vi "test.vi"() -> ()   [LabVIEW 2020]
uses:
  <vilib>/rvi/Emulation/niFpgaGetClockAttributes.vi
  <vilib>/rvi/Emulation/niFpgaSctlEmulationGetInTimedLoop.vi
  <vilib>/rvi/Emulation/niFpgaEmulationReportErrorSimple.vi
  <vilib>/rvi/DataTransferAndStorage/Container/Common/niFpgaContainerExecOnDevCompGetState.vi
  <vilib>/rvi/Emulation/niFpgaEmulationIsFPGAContextNoSignature.vi
  <vilib>/rvi/DataTransferAndStorage/Container/Common/niFpgaContainerGetUniqueNameForEmu.vi
  <vilib>/rvi/Memory/Memory_Emulation/niFpgaMemoryEmulationCacheClearOnFirstRun.vi
  <vilib>/rvi/Memory/Memory_Emulation/nirvimemoryEmulationManagerCache_MakeExclusive.vi
  <vilib>/rvi/Memory/Memory_Emulation/niFpgaMemoryEmulationValidateCache.vi
  <vilib>/rvi/Memory/Memory_Emulation/nirvimemoryEmulationManagerCache_InsertValue.vi
  <vilib>/Utility/error.llb/Clear Errors.vi
  <vilib>/rvi/Memory/Memory_Emulation/nirvimemoryEmulationManagerCache_ReleaseExclusive.vi
  <vilib>/rvi/Memory/Memory_Emulation/nirvimemoryEmulationManagerCache_GetValue.vi
  <vilib>/rvi/Memory/Memory_Emulation/nirvimemoryEmulationManagerCache_SetValue.vi
  <vilib>/rvi/Emulation/niFpgaProcessEmulError.vi
  <vilib>/rvi/DataTransferAndStorage/Container/Common/niFpgaContainerSetEmuInfo.vi
  <vilib>/rvi/eio/common/nirviEmuReportErrorAndStop.vi
  <vilib>/rvi/interface/RandomDataEmulation/niFpgaRandomDataHandleErrors.vi
  <vilib>/rvi/errors/niFpgaSetErrorForExecOnDevCompSimple.vi
  <vilib>/rvi/FIFO/Fifo_Resource/nirvififoEmulationSetSize.vi
  <vilib>/rvi/FIFO/Fifo_Resource/nirviFifoEmulationQueueMgr.vi
  <instcachedir>/0/nirviFifoEmulationQueueMgr_E5CAEC123FF24DC58D834DCA3CDAA9B5.lvgen/nirviFifoEmulationQueueMgr_E5CAEC123FF24DC58D834DCA3CDAA9B5_004.vi
  <vilib>/rvi/FIFO/Fifo_Resource/nirvififoEmulationDetermineInputValidOut.vi
  <vilib>/rvi/FIFO/Fifo_Resource/nirvififoEmulationCreateLock.vi
  <vilib>/rvi/FIFO/Fifo_Resource/nirvififoEmulationObtainLock.vi
  <vilib>/rvi/FIFO/Fifo_Resource/nirvififoEmulationReleaseLock.vi
  <vilib>/rvi/occurrence/nirviWaitOnOccurrenceBase.vi
  <vilib>/rvi/errors/nirviReportUnexpectedCaseInternalError.vi
  <vilib>/rvi/errors/nirviReportUnexpectedCaseInternalError (U32).vi
  <vilib>/rvi/Emulation/niFpgaSctlEmulationResourceMgr.vi
  <vilib>/rvi/Emulation/niFpgaCriticalErrorInLSC.vi
  <vilib>/rvi/DataTransferAndStorage/Container/XNode/niFpgaContainer.xnode
  <vilib>/rvi/DataTransferAndStorage/Register/Emulation/niFpgaRegisterEmulationRefIn.vi
  <vilib>/rvi/LocalResourceManager/LocalResourceManager.xnode
  <vilib>/rvi/interface/RandomDataEmulation/nirviRandomDataFpgaReadWriteTemplate.vi
  <vilib>/rvi/FIFO/Fifo_Resource/niFpgaFifoEmulationRefIn.vi
  <vilib>/rvi/Memory/Memory_Emulation/niFpgaMemoryEmulationRefIn.vi
  <vilib>/eio/EIONode/EIONode.xnode
  <vilib>/rvi/eio/common/nirviEmuTemplateMethod_errors.vi
panel:
  out "Actual loop rate (ticks) 3":u32
  out "Timed Out? 4":bool
  out "Mod1/AI0 4":fxp<+/-,32,16>
  out "data read iteration":i32
  out "Actual loop rate (ticks) 2":u32
  out "Timed Out? 3":bool
  out "Mod1/AI0 3":fxp<+/-,32,16>
  out "array w/ subset deleted 2":fxp<+/-,32,16>[](array[numeric])
  out "fixed-point":fxp<+/-,32,16>
  out "fixed-point 2":fxp<+/-,32,16>
  out "loop number":i32
  out "x > y?":bool
  in  "stop target":bool
  out "array w/ subset deleted":fxp<+/-,32,16>[](array[numeric])
  out "y(MLP1)":fxp<+/-,32,16>
  out "y(MLP2)":fxp<+/-,32,16>
  out "Timed Out? 2":bool
  out "Mod1/AI0 2":fxp<+/-,32,16>
  out "Actual loop rate (ticks)":u32
  out "Timed Out?":bool
  out "Mod1/AI0":fxp<+/-,32,16>
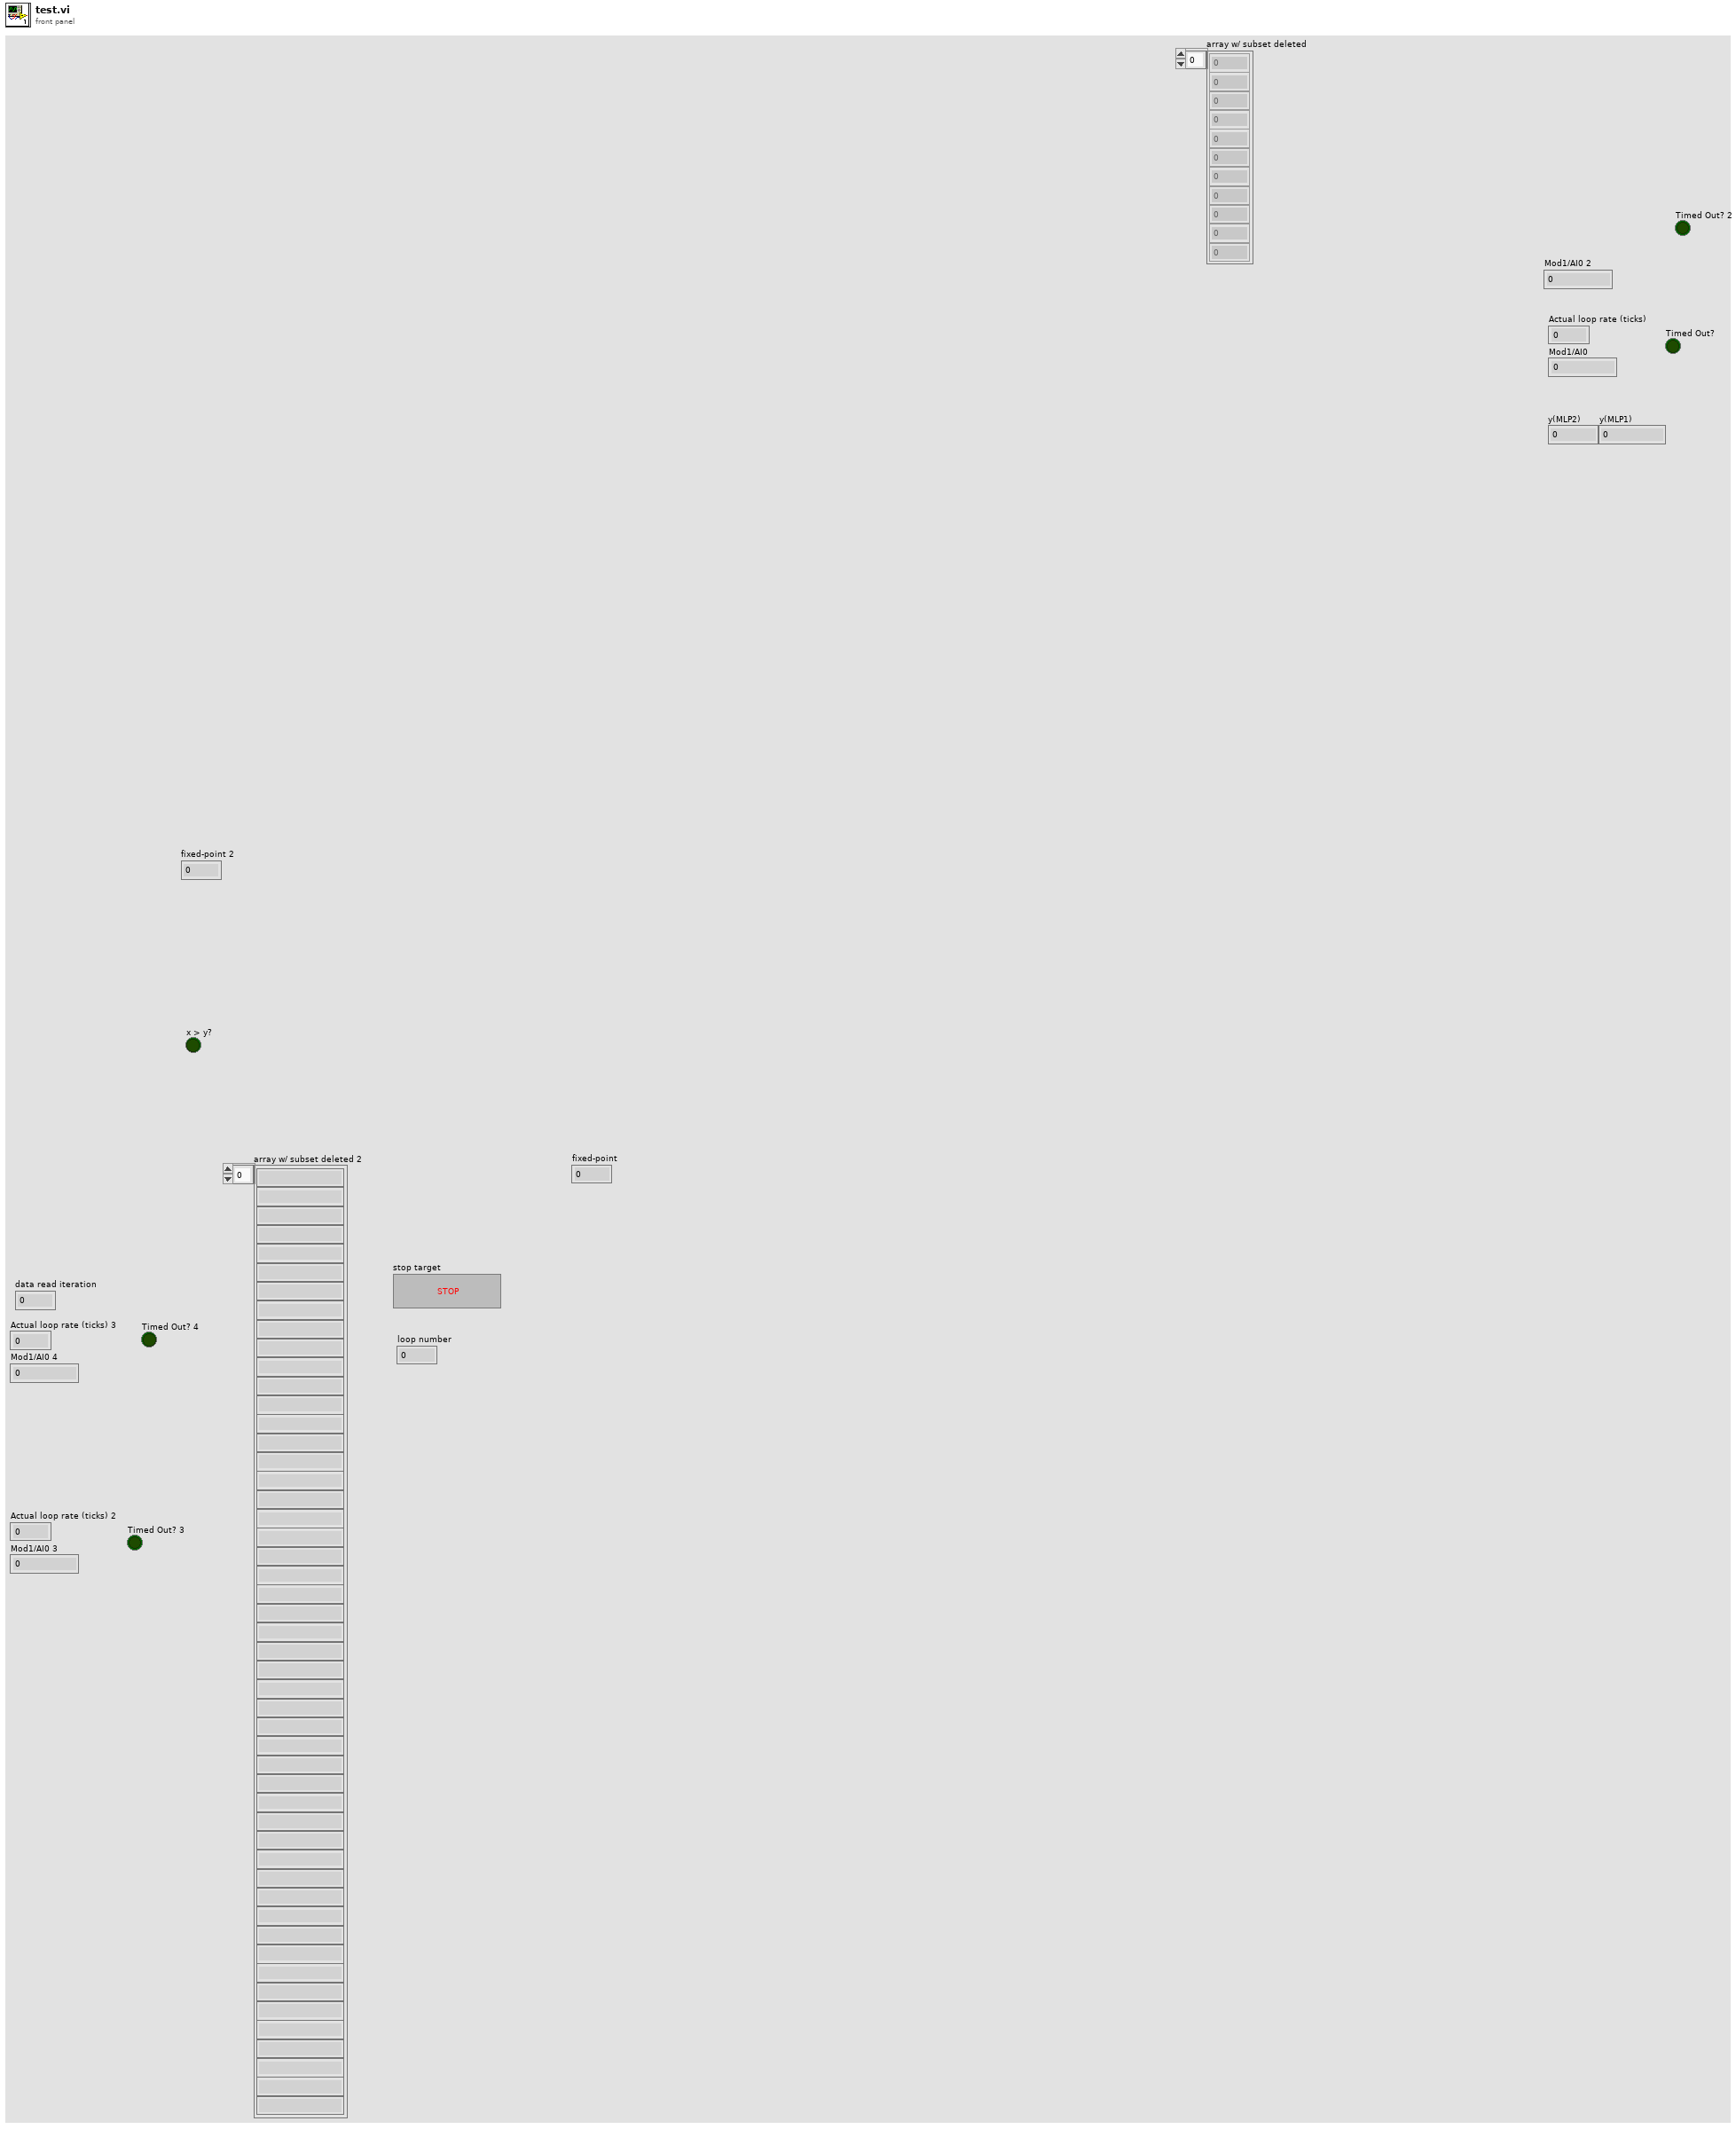
[diagram p1: front panel]
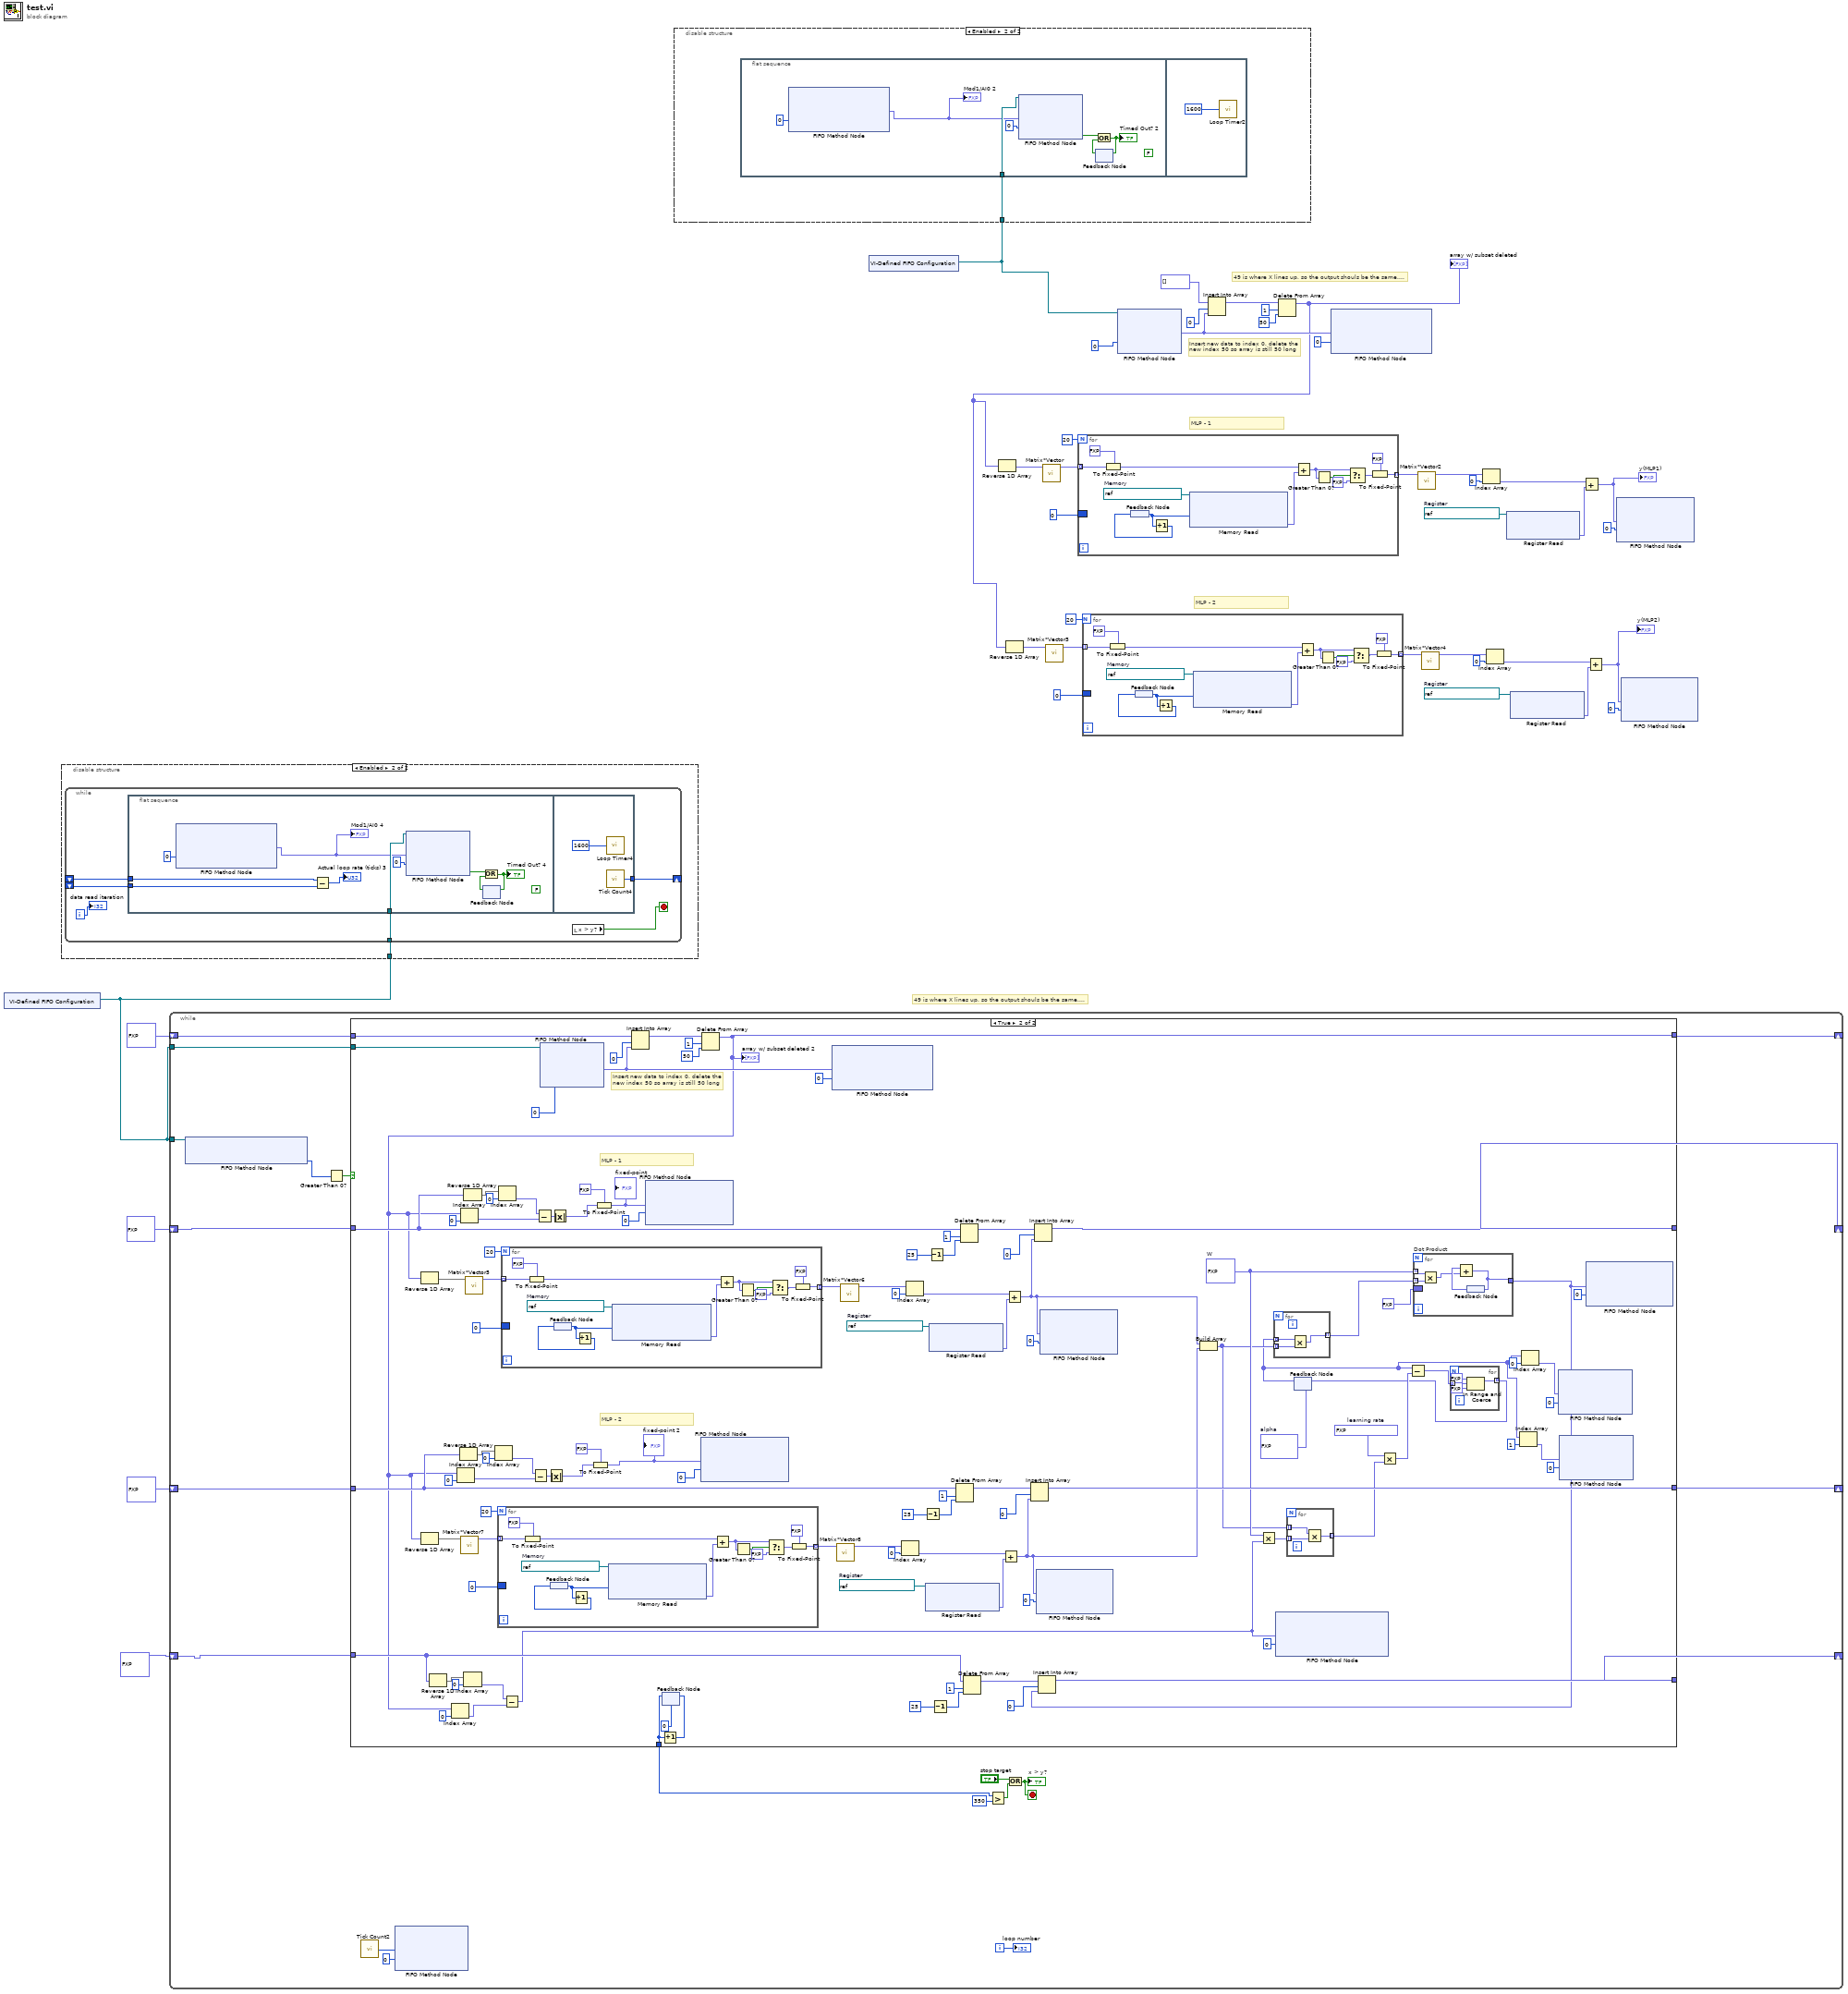
[diagram p0: block diagram]
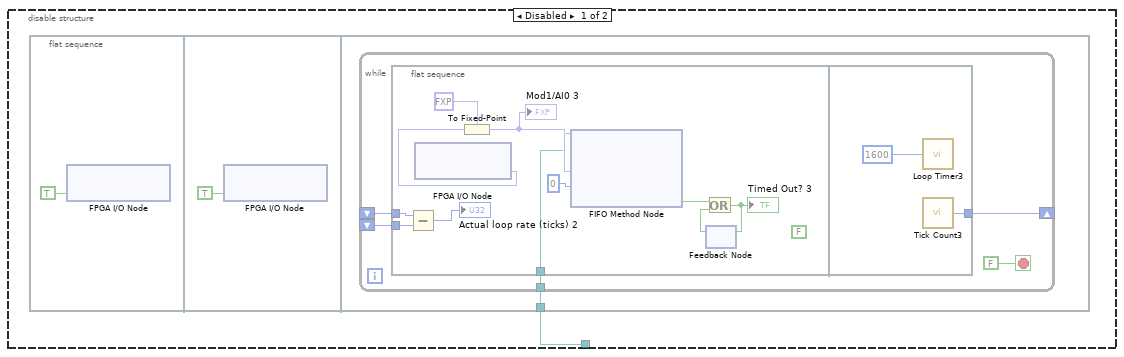
[diagram p2: hidden frame]
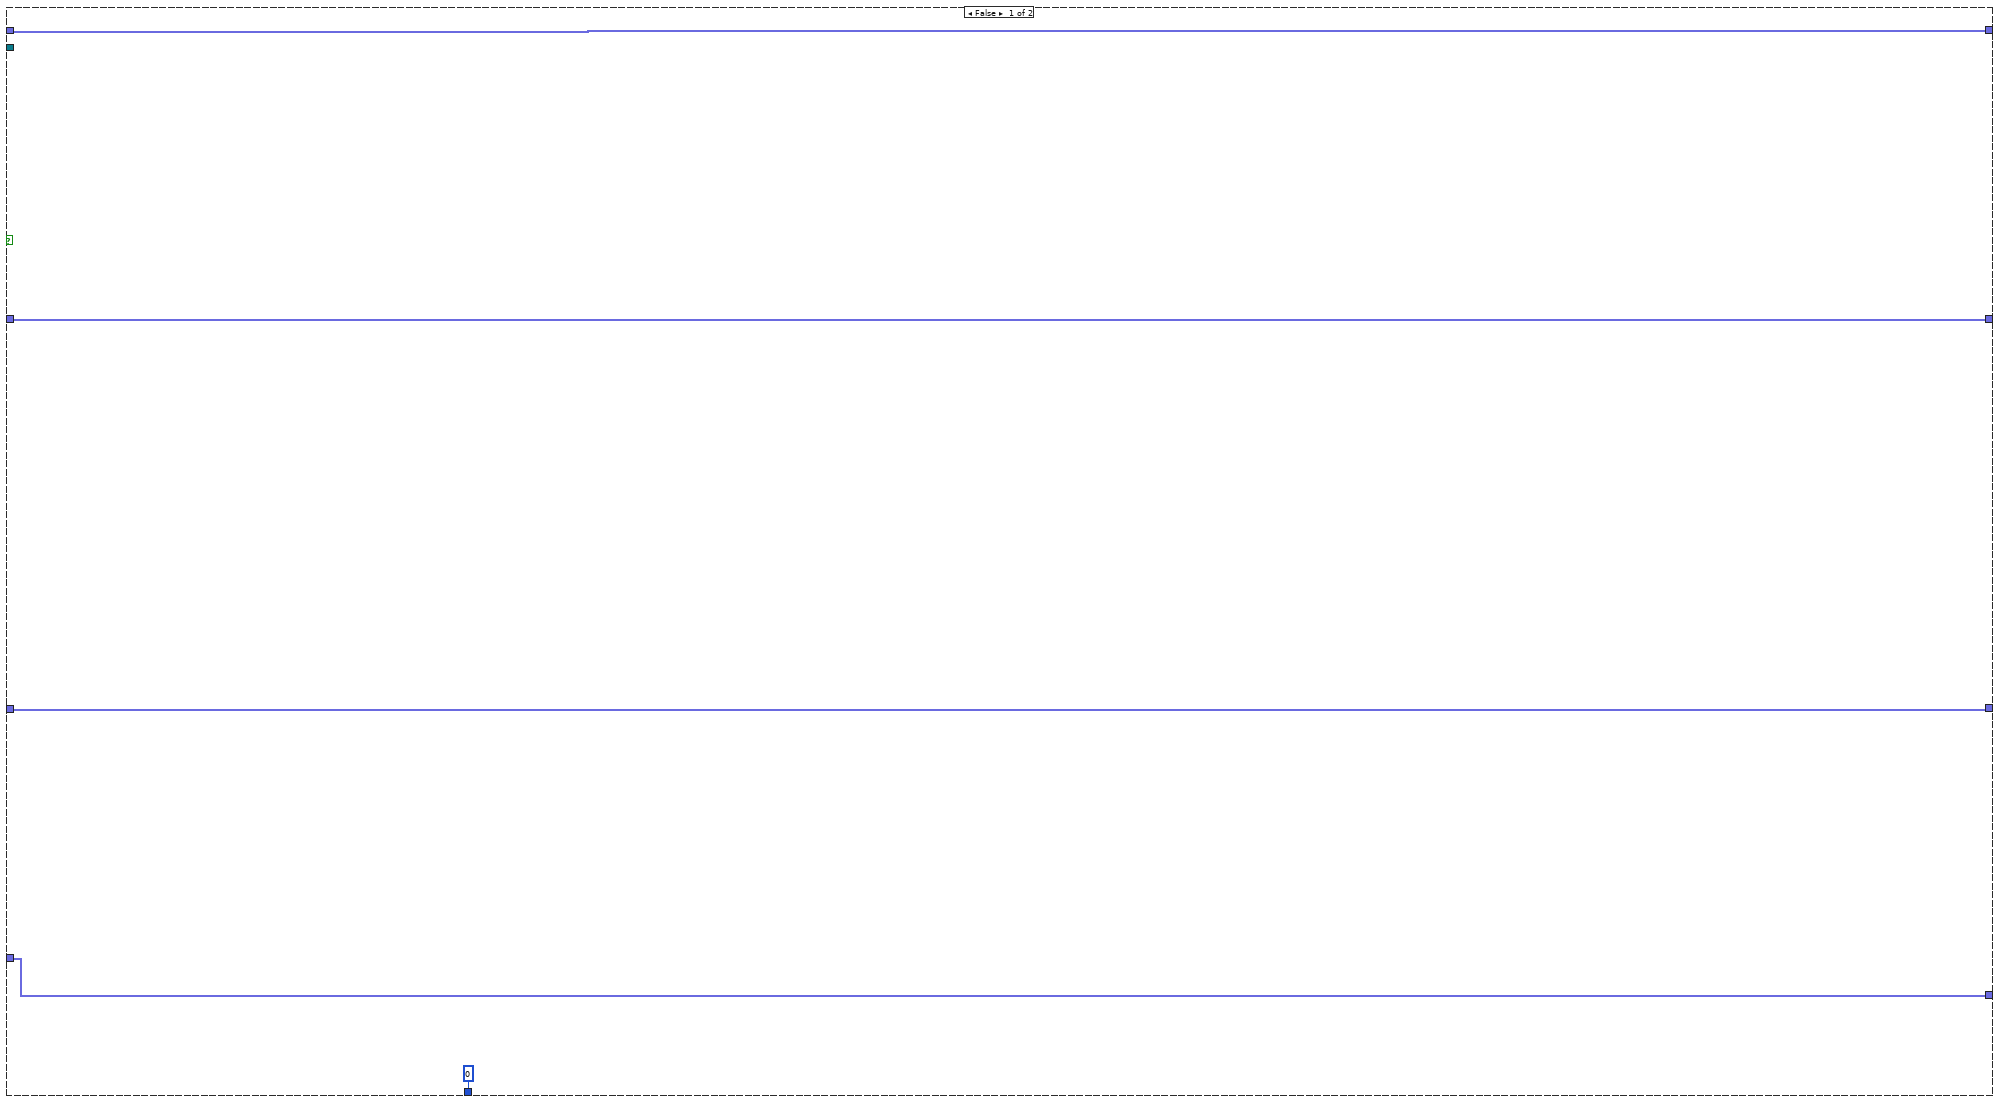
[diagram p3: hidden frame]
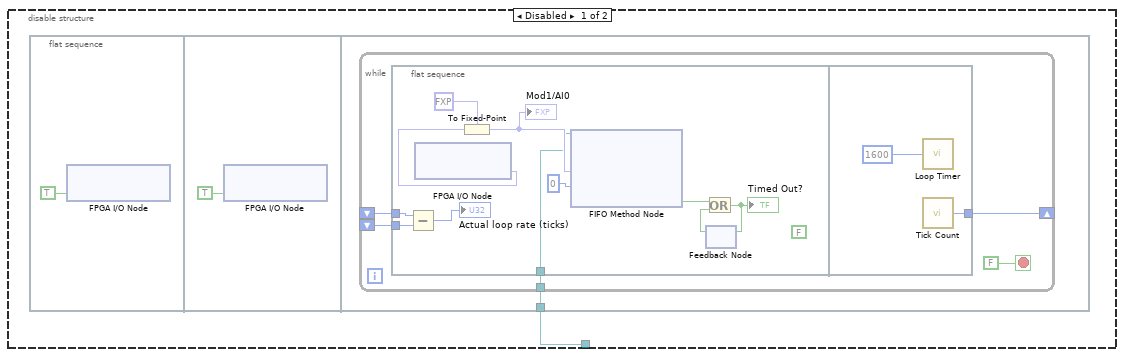
[diagram p4: hidden frame]
diagram:
  w22 = refnum<k21> "Register-MLP_2_B_1"  # Register
  w34 = refnum<k21> "Register-MLP_1_B_1"  # Register
  # "49 is where X lines up, so the output shouls be the same...."
  # "Insert new data to index 0, delete the\nnew index 50 so array is still 50 long"
  # "MLP - 2"
  # "MLP - 1"
  # "49 is where X lines up, so the output shouls be the same...."
  n1 = xnode "VI-Defined FIFO Configuration"() -> ("FIFO Out"=w1:refnum<k21>)
  n2 = disable-structure shown="Enabled" {
    disable-tunnel: w1 -> [w40 w62]
    frame Disabled {
      n3 = flat-sequence {
        tunnel: w40 -> [w43]
        frame #0 {
          n4 = xnode "FPGA I/O Node"("Mod1/Stop"=TRUE) -> ()  [unwired: 1 in, 1 out]
        }
        frame #1 {
          n5 = xnode "FPGA I/O Node"("Mod1/Start"=TRUE) -> ()  [unwired: 1 in, 1 out]
        }
        frame #2 {
          n6 = while {
            shift-right: [w48] -> _
            shift-left: _ -> [w47]
            shift-left: _ -> [w46]
            tunnel: w43 -> [w44]
            stop <- FALSE stop-if-true
            n7 = flat-sequence {
              tunnel: w47 -> [w59]
              tunnel: w46 -> [w58]
              tunnel: w44 -> [w49]
              tunnel: [w61] -> w48
              frame #0 {
                (unwired) FALSE
                n8 = Subtract(x=w59, y=w58) -> (x-y=→"Actual loop rate (ticks) 2":u32)
                n9 = xnode "FPGA I/O Node"() -> ("Mod1/AI0"=w51:fxp<+/-,24,7>)  [unwired: 1 in, 1 out]
                n10 = To Fixed-Point(fixed-point type=fxp<+/-,32,16> 0.0 ("f"), number=w51) -> (fixed-point=w50:fxp<+/-,32,16>)
                "Mod1/AI0 3" <- w50
                n11 = xnode ("FIFO Method Node")("Element"=w50, "Timeout"=0, "FIFO In"=w49) -> ("Timed Out?"=w55:bool)  [unwired: 1 in, 2 out]
                n12 = feedback #1() -> (w54:bool)  [unwired: 1 in]
                n13 = Or(x=w55, y=w54) -> (x .or. y?=w53:bool)
                "Timed Out? 3" <- w53
                n14 = feedback-in #1(w53) -> ()
              }
              frame #1 {
                n15 = call "Loop Timer3"("Count(Ticks)"=u32 1600 ("Rate (uSec)")) -> ()  [unwired: 1 out]
                n16 = call "Tick Count3"() -> ("Tick Count(Ticks)"=w61:u32)
              }
            }
          }
        }
      }
    }
    frame Enabled {
      n17 = while {
        shift-right: [w68] -> _
        shift-left: _ -> [w67]
        shift-left: _ -> [w66]
        tunnel: w62 -> [w65]
        i -> [w64]
        stop <- w63 stop-if-true
        n18 = flat-sequence {
          tunnel: w67 -> [w78]
          tunnel: w66 -> [w77]
          tunnel: w65 -> [w71]
          tunnel: [w80] -> w68
          frame #0 {
            (unwired) FALSE
            n19 = xnode ("FIFO Method Node")("Timeout"=0) -> ("Element"=w70:fxp<+/-,32,16>)  [unwired: 1 in, 2 out]
            "Mod1/AI0 4" <- w70
            n20 = Subtract(x=w78, y=w77) -> (x-y=→"Actual loop rate (ticks) 3":u32)
            n21 = xnode ("FIFO Method Node")("Element"=w70, "Timeout"=0, "FIFO In"=w71) -> ("Timed Out?"=w74:bool)  [unwired: 1 in, 2 out]
            n22 = feedback #2() -> (w73:bool)  [unwired: 1 in]
            n23 = Or(x=w74, y=w73) -> (x .or. y?=w72:bool)
            "Timed Out? 4" <- w72
            n24 = feedback-in #2(w72) -> ()
          }
          frame #1 {
            n25 = call "Loop Timer4"("Count(Ticks)"=u32 1600 ("Rate (uSec)")) -> ()  [unwired: 1 out]
            n26 = call "Tick Count4"() -> ("Tick Count(Ticks)"=w80:u32)
          }
        }
        n27 = local read "x > y?"() -> (w63:bool)
        "data read iteration" <- w64
      }
    }
  }
  n28 = while {
    shift-right: [w97] -> _
    shift-left: fxp<+/-,32,16>[] [0.0, 0.0, 0.0, 0.0, 0.0, 0.0, 0.0, 0.0, 0.0, 0.0, 0.0, 0.0, 0.0, 0.0, 0.0, 0.0, 0.0, 0.0, 0.0, 0.0, 0.0, 0.0, 0.0, 0.0, 0.0, 0.0, 0.0, 0.0, 0.0, 0.0, 0.0, 0.0, 0.0, 0.0, 0.0, 0.0, 0.0, 0.0, 0.0, 0.0, 0.0, 0.0, 0.0, 0.0, 0.0, 0.0, 0.0, 0.0, 0.0, 0.0] -> [w100]
    shift-right: [w98] -> _
    shift-left: fxp<+/-,32,16>[] [0.0, 0.0, 0.0, 0.0, 0.0, 0.0, 0.0, 0.0, 0.0, 0.0, 0.0, 0.0, 0.0, 0.0, 0.0, 0.0, 0.0, 0.0, 0.0, 0.0, 0.0, 0.0, 0.0, 0.0, 0.0] -> [w99]
    tunnel: w1 -> [w93]
    tunnel: w1 -> [w92]
    shift-right: [w88] -> _
    shift-left: fxp<+/-,32,16>[] [0.0, 0.0, 0.0, 0.0, 0.0, 0.0, 0.0, 0.0, 0.0, 0.0, 0.0, 0.0, 0.0, 0.0, 0.0, 0.0, 0.0, 0.0, 0.0, 0.0, 0.0, 0.0, 0.0, 0.0, 0.0] -> [w89]
    shift-right: [w87] -> _
    shift-left: fxp<+/-,32,16>[] [0.0, 0.0, 0.0, 0.0, 0.0, 0.0, 0.0, 0.0, 0.0, 0.0, 0.0, 0.0, 0.0, 0.0, 0.0, 0.0, 0.0, 0.0, 0.0, 0.0, 0.0, 0.0, 0.0, 0.0, 0.0] -> [w86]
    i -> [w94]
    stop <- w81 stop-if-true
    n29 = xnode ("FIFO Method Node")("FIFO In"=w93) -> ("Number of Elements to Read"=w96:u32)  [unwired: 1 in, 2 out]
    n30 = Greater Than 0?(x=w96) -> (x > 0?=w95:bool)
    n31 = case shown="True" w95 {
      tunnel: w100 -> [w105 w154]
      tunnel: w99 -> [w104 w198]
      tunnel: [w104 w196] -> w98
      tunnel: [w105 w106] -> w97
      tunnel: w92 -> [_ w183]
      tunnel: w89 -> [w103 w156]
      tunnel: [w103 w155] -> w88
      tunnel: w86 -> [w102 w136]
      tunnel: [w102 w139] -> w87
      tunnel: [0 ("length") w121] -> w85
      frame False {
      }
      frame True {
        w128 = fxp<+/-,32,16> 0.0001068115234375  # learning rate
        w131 = fxp<+/-,32,16>[] [1.0, 1.0]  # W
        w127 = fxp<+/-,32,16>[] [0.5, 0.5]  # alpha
        w175 = refnum<k21> "Register-MLP_2_B_1"  # Register
        w204 = refnum<k21> "Register-MLP_1_B_1"  # Register
        # "Insert new data to index 0, delete the\nnew index 50 so array is still 50 long"
        # "MLP - 2"
        # "MLP - 1"
        n32 = Reverse 1D Array(array=w136) -> (reversed array=w138:fxp<+/-,32,16>[])
        n33 = Reverse 1D Array(array=w156) -> (reversed array=w158:fxp<+/-,32,16>[])
        n34 = Reverse 1D Array(array=w198) -> (reversed array=w186:fxp<+/-,32,16>[])
        n35 = Index Array(array=w138, index=0) -> (element=w134:fxp<+/-,32,16>)
        n36 = Index Array(array=w158, index=0) -> (element=w159:fxp<+/-,32,16>)
        n37 = Index Array(array=w186, index=0) -> (element=w187:fxp<+/-,32,16>)
        n38 = xnode ("FIFO Method Node")("Timeout"=0, "FIFO In"=w183) -> ("Element"=w182:fxp<+/-,32,16>)  [unwired: 1 in, 3 out]
        n39 = Insert Into Array(array=w154, index=0, new element=w182) -> (w152:fxp<+/-,32,16>[])
        n40 = feedback #3(0 ("length")) -> (w121:i32)
        n41 = Increment(x=w121) -> (x+1=w122:i32)
        n42 = feedback-in #3(w122) -> ()
        n43 = Delete From Array(array=w152, length=1, index=50) -> (array with subset deleted=w106:fxp<+/-,32,16>[])  [unwired: 1 out]
        "array w/ subset deleted 2" <- w106
        n44 = Reverse 1D Array(array=w106) -> (reversed array=w150:fxp<+/-,32,16>[])
        n45 = Reverse 1D Array(array=w106) -> (reversed array=w149:fxp<+/-,32,16>[])
        n46 = Index Array(array=w106, index=0) -> (element=w133:fxp<+/-,32,16>)
        n47 = Index Array(array=w106, index=0) -> (element=w170:fxp<+/-,32,16>)
        n48 = call "Matrix*Vector7"("Vector b"=w149) -> ("Vector c"=w178:fxp<+/-,64,38>[])  [unwired: 10 in]
        n49 = Index Array(array=w106, index=0) -> (element=w199:fxp<+/-,32,16>)
        n50 = call "Matrix*Vector5"("Vector b"=w150) -> ("Vector c"=w207:fxp<+/-,64,38>[])  [unwired: 10 in]
        n51 = for {
          N: 20 -> [_]
          tunnel: w178 -> [w229] mode=indexing
          tunnel: [w226] -> w177 mode=indexing
          border: u32 0 ("Timeout") -> [_]
          w233 = refnum<k21> "Memory-MLP_2_B_0"  # Memory
          n52 = To Fixed-Point(fixed-point type=fxp<+/-,32,16> 0.0 ("f"), number=w229) -> (fixed-point=w234:fxp<+/-,32,16>)
          n53 = feedback #4() -> (w232:u32)
          n54 = Increment(x=w232) -> (x+1=w231:u32)
          n55 = feedback-in #4(w231) -> ()
          n56 = xnode ("Memory Read")("Address"=w232, "Memory In"=w233) -> ("Data"=w230:fxp<+/-,32,16>)  [unwired: 1 out]
          n57 = Add(x=w234, y=w230) -> (x+y=w236:fxp<+/-,33,17>)
          n58 = Greater Than 0?(x=w236) -> (x > 0?=w238:bool)
          n59 = Select(t=w236, s=w238, f=fxp<+/-,33,17> 0.0) -> (s? t:f=w227:fxp<+/-,33,17>)
          n60 = To Fixed-Point(fixed-point type=fxp<+/-,32,16> 0.0 ("f"), number=w227) -> (fixed-point=w226:fxp<+/-,32,16>)
        }
        n61 = for {
          N: 20 -> [_]
          tunnel: w207 -> [w242] mode=indexing
          tunnel: [w239] -> w206 mode=indexing
          border: u32 0 ("Timeout") -> [_]
          w246 = refnum<k21> "Memory-MLP_1_B_0"  # Memory
          n62 = To Fixed-Point(fixed-point type=fxp<+/-,32,16> 0.0 ("f"), number=w242) -> (fixed-point=w247:fxp<+/-,32,16>)
          n63 = feedback #5() -> (w245:u32)
          n64 = Increment(x=w245) -> (x+1=w244:u32)
          n65 = feedback-in #5(w244) -> ()
          n66 = xnode ("Memory Read")("Address"=w245, "Memory In"=w246) -> ("Data"=w243:fxp<+/-,32,16>)  [unwired: 1 out]
          n67 = Add(x=w247, y=w243) -> (x+y=w249:fxp<+/-,33,17>)
          n68 = Greater Than 0?(x=w249) -> (x > 0?=w251:bool)
          n69 = Select(t=w249, s=w251, f=fxp<+/-,33,17> 0.0) -> (s? t:f=w240:fxp<+/-,33,17>)
          n70 = To Fixed-Point(fixed-point type=fxp<+/-,32,16> 0.0 ("f"), number=w240) -> (fixed-point=w239:fxp<+/-,32,16>)
        }
        n71 = Subtract(x=w134, y=w133) -> (x-y=w117:fxp<+/-,32,16>)
        n72 = Subtract(x=w159, y=w170) -> (x-y=w160:fxp<+/-,33,17>)
        n73 = Subtract(x=w187, y=w199) -> (x-y=w188:fxp<+/-,33,17>)
        n74 = Absolute Value(x=w160) -> (abs(x)=w162:fxp<+,32,16>)
        n75 = Absolute Value(x=w188) -> (abs(x)=w189:fxp<+,32,16>)
        n76 = To Fixed-Point(fixed-point type=fxp<+/-,32,16> 0.0 ("f"), number=w162) -> (fixed-point=w161:fxp<+/-,32,16>)
        "fixed-point 2" <- w161
        n77 = To Fixed-Point(fixed-point type=fxp<+/-,32,16> 0.0 ("f"), number=w189) -> (fixed-point=w115:fxp<+/-,32,16>)
        "fixed-point" <- w115
        n78 = xnode ("FIFO Method Node")("Element"=w115, "Timeout"=0) -> ()  [unwired: 1 in, 2 out]
        n79 = xnode ("FIFO Method Node")("Element"=w161, "Timeout"=0) -> ()  [unwired: 1 in, 2 out]
        n80 = xnode ("FIFO Method Node")("Element"=w182, "Timeout"=0) -> ()  [unwired: 1 in, 2 out]
        n81 = call "Matrix*Vector8"("Vector b"=w177) -> ("Vector c"=w180:fxp<+/-,64,37>[])  [unwired: 10 in]
        n82 = call "Matrix*Vector6"("Vector b"=w206) -> ("Vector c"=w209:fxp<+/-,64,37>[])  [unwired: 10 in]
        n83 = Index Array(array=w180, index=0) -> (element=w147:fxp<+/-,64,37>)
        n84 = Index Array(array=w209, index=0) -> (element=w148:fxp<+/-,64,37>)
        n85 = Decrement(x=25) -> (x-1=w168:i32)
        n86 = xnode ("Register Read")("Register In"=w175) -> ("Data"=w174:fxp<+/-,32,16>)  [unwired: 1 out]
        n87 = Decrement(x=25) -> (x-1=w195:i32)
        n88 = xnode ("Register Read")("Register In"=w204) -> ("Data"=w203:fxp<+/-,32,16>)  [unwired: 1 out]
        n89 = Decrement(x=25) -> (x-1=w143:i32)
        n90 = Delete From Array(array=w156, length=1, index=w168) -> (array with subset deleted=w166:fxp<+/-,32,16>[])  [unwired: 1 out]
        n91 = Delete From Array(array=w198, length=1, index=w195) -> (array with subset deleted=w193:fxp<+/-,32,16>[])  [unwired: 1 out]
        n92 = Delete From Array(array=w136, length=1, index=w143) -> (array with subset deleted=w141:fxp<+/-,32,16>[])  [unwired: 1 out]
        n93 = Add(x=w147, y=w174) -> (x+y=w146:fxp<+/-,32,16>)
        n94 = Add(x=w148, y=w203) -> (x+y=w145:fxp<+/-,32,16>)
        n95 = Insert Into Array(array=w166, index=0, new element=w146) -> (w155:fxp<+/-,32,16>[])
        n96 = Insert Into Array(array=w193, index=0, new element=w145) -> (w196:fxp<+/-,32,16>[])
        n97 = xnode ("FIFO Method Node")("Element"=w146, "Timeout"=0) -> ()  [unwired: 1 in, 2 out]
        n98 = xnode ("FIFO Method Node")("Element"=w145, "Timeout"=0) -> ()  [unwired: 1 in, 2 out]
        n99 = Build Array(w145, w146) -> (w125:fxp<+/-,32,16>[])
        n100 = Multiply(x=w131, y=w117) -> (x*y=w126:fxp<+/-,32,16>[])
        n101 = xnode ("FIFO Method Node")("Element"=w117, "Timeout"=0) -> ()  [unwired: 1 in, 2 out]
        n102 = for {
          tunnel: [w220] -> w129 mode=indexing
          tunnel: w125 -> [w219] mode=indexing
          tunnel: w126 -> [w218] mode=indexing
          n103 = Multiply(x=w219, y=w218) -> (x*y=w220:fxp<+/-,64,32>)
        }
        n104 = feedback #6(w127) -> (w118:fxp<+/-,32,16>[])
        n105 = for {
          tunnel: [w217] -> w132 mode=indexing
          tunnel: w118 -> [w216] mode=indexing
          tunnel: w125 -> [w215] mode=indexing
          n106 = Multiply(x=w216, y=w215) -> (x*y=w217:fxp<+/-,32,16>)
        }
        n107 = Multiply(x=w128, y=w129) -> (x*y=w130:fxp<+/-,32,16>[])
        n108 = Subtract(x=w118, y=w130) -> (x-y=w109:fxp<+/-,32,16>[])
        n109 = for "Dot Product" {
          tunnel: [w224] -> w114
          tunnel: w132 -> [w223] mode=indexing
          tunnel: w131 -> [w222] mode=indexing
          border: fxp<+/-,32,16> 0.0 -> [_]
          n110 = Multiply(x=w222, y=w223) -> (x*y=w221:fxp<+/-,32,16>)
          n111 = feedback #7() -> (w225:fxp<+/-,32,16>)
          n112 = Add(x=w225, y=w221) -> (x+y=w224:fxp<+/-,32,16>)
          n113 = feedback-in #7(w224) -> ()
        }
        n114 = Insert Into Array(array=w141, index=0, new element=w114) -> (w139:fxp<+/-,32,16>[])
        n115 = for {
          tunnel: w109 -> [w214] mode=indexing
          tunnel: [w211] -> w108 mode=indexing
          n116 = In Range and Coerce(upper limit=fxp<+/-,32,16> 1.0, x=w214, lower limit=fxp<+/-,32,16> 0.0) -> (coerced(x)=w211:fxp<+/-,32,16>)  [unwired: 1 out]
        }
        n117 = feedback-in #6(w108) -> ()
        n118 = Index Array(array=w118, index=1) -> (element=w110:fxp<+/-,32,16>)
        n119 = Index Array(array=w118, index=0) -> (element=w113:fxp<+/-,32,16>)
        n120 = xnode ("FIFO Method Node")("Element"=w113, "Timeout"=0) -> ()  [unwired: 1 in, 2 out]
        n121 = xnode ("FIFO Method Node")("Element"=w110, "Timeout"=0) -> ()  [unwired: 1 in, 2 out]
        n122 = xnode ("FIFO Method Node")("Element"=w114, "Timeout"=0) -> ()  [unwired: 1 in, 2 out]
      }
    }
    n123 = call "Tick Count2"() -> ("Tick Count(Ticks)"=w91:u32)
    n124 = xnode ("FIFO Method Node")("Element"=w91, "Timeout"=0) -> ()  [unwired: 1 in, 2 out]
    n125 = Greater?(x=w85, y=350) -> (0:w82:bool)
    n126 = Or(x="stop target", y=w82) -> (x .or. y?=w81:bool)
    "x > y?" <- w81
    "loop number" <- w94
  }
  n127 = xnode "VI-Defined FIFO Configuration"() -> ("FIFO Out"=w10:refnum<k21>)
  n128 = disable-structure shown="Enabled" {
    disable-tunnel: w10 -> [w252 w274]
    frame Disabled {
      n129 = flat-sequence {
        tunnel: w252 -> [w255]
        frame #0 {
          n130 = xnode "FPGA I/O Node"("Mod1/Stop"=TRUE) -> ()  [unwired: 1 in, 1 out]
        }
        frame #1 {
          n131 = xnode "FPGA I/O Node"("Mod1/Start"=TRUE) -> ()  [unwired: 1 in, 1 out]
        }
        frame #2 {
          n132 = while {
            shift-right: [w260] -> _
            shift-left: _ -> [w259]
            shift-left: _ -> [w258]
            tunnel: w255 -> [w256]
            stop <- FALSE stop-if-true
            n133 = flat-sequence {
              tunnel: w259 -> [w271]
              tunnel: w258 -> [w270]
              tunnel: w256 -> [w261]
              tunnel: [w273] -> w260
              frame #0 {
                (unwired) FALSE
                n134 = Subtract(x=w271, y=w270) -> (x-y=→"Actual loop rate (ticks)":u32)
                n135 = xnode "FPGA I/O Node"() -> ("Mod1/AI0"=w263:fxp<+/-,24,7>)  [unwired: 1 in, 1 out]
                n136 = To Fixed-Point(fixed-point type=fxp<+/-,32,16> 0.0 ("f"), number=w263) -> (fixed-point=w262:fxp<+/-,32,16>)
                "Mod1/AI0" <- w262
                n137 = xnode ("FIFO Method Node")("Element"=w262, "Timeout"=0, "FIFO In"=w261) -> ("Timed Out?"=w267:bool)  [unwired: 1 in, 2 out]
                n138 = feedback #8() -> (w266:bool)  [unwired: 1 in]
                n139 = Or(x=w267, y=w266) -> (x .or. y?=w265:bool)
                "Timed Out?" <- w265
                n140 = feedback-in #8(w265) -> ()
              }
              frame #1 {
                n141 = call "Loop Timer"("Count(Ticks)"=u32 1600 ("Rate (uSec)")) -> ()  [unwired: 1 out]
                n142 = call "Tick Count"() -> ("Tick Count(Ticks)"=w273:u32)
              }
            }
          }
        }
      }
    }
    frame Enabled {
      n143 = flat-sequence {
        tunnel: w274 -> [w277]
        frame #0 {
          (unwired) FALSE
          n144 = xnode ("FIFO Method Node")("Timeout"=0) -> ("Element"=w276:fxp<+/-,32,16>)  [unwired: 1 in, 2 out]
          "Mod1/AI0 2" <- w276
          n145 = xnode ("FIFO Method Node")("Element"=w276, "Timeout"=0, "FIFO In"=w277) -> ("Timed Out?"=w280:bool)  [unwired: 1 in, 2 out]
          n146 = feedback #9() -> (w279:bool)  [unwired: 1 in]
          n147 = Or(x=w280, y=w279) -> (x .or. y?=w278:bool)
          "Timed Out? 2" <- w278
          n148 = feedback-in #9(w278) -> ()
        }
        frame #1 {
          n149 = call "Loop Timer2"("Count(Ticks)"=u32 1600 ("Rate (uSec)")) -> ()  [unwired: 1 out]
        }
      }
    }
  }
  n150 = xnode ("FIFO Method Node")("Timeout"=0, "FIFO In"=w10) -> ("Element"=w29:fxp<+/-,32,16>)  [unwired: 1 in, 3 out]
  n151 = Insert Into Array(array=fxp<+/-,32,16>[] [], index=0, new element=w29) -> (w17:fxp<+/-,32,16>[])
  n152 = Delete From Array(array=w17, length=1, index=50) -> (array with subset deleted=w11:fxp<+/-,32,16>[])  [unwired: 1 out]
  "array w/ subset deleted" <- w11
  n153 = Reverse 1D Array(array=w11) -> (reversed array=w15:fxp<+/-,32,16>[])
  n154 = Reverse 1D Array(array=w11) -> (reversed array=w14:fxp<+/-,32,16>[])
  n155 = call "Matrix*Vector"("Vector b"=w15) -> ("Vector c"=w36:fxp<+/-,64,38>[])  [unwired: 10 in]
  n156 = call "Matrix*Vector3"("Vector b"=w14) -> ("Vector c"=w25:fxp<+/-,64,38>[])  [unwired: 10 in]
  n157 = for {
    N: 20 -> [_]
    tunnel: w36 -> [w286] mode=indexing
    tunnel: [w283] -> w6 mode=indexing
    border: u32 0 ("Timeout") -> [_]
    w290 = refnum<k21> "Memory-MLP_1_B_0"  # Memory
    n158 = To Fixed-Point(fixed-point type=fxp<+/-,32,16> 0.0 ("f"), number=w286) -> (fixed-point=w291:fxp<+/-,32,16>)
    n159 = feedback #10() -> (w289:u32)
    n160 = Increment(x=w289) -> (x+1=w288:u32)
    n161 = feedback-in #10(w288) -> ()
    n162 = xnode ("Memory Read")("Address"=w289, "Memory In"=w290) -> ("Data"=w287:fxp<+/-,32,16>)  [unwired: 1 out]
    n163 = Add(x=w291, y=w287) -> (x+y=w293:fxp<+/-,33,17>)
    n164 = Greater Than 0?(x=w293) -> (x > 0?=w295:bool)
    n165 = Select(t=w293, s=w295, f=fxp<+/-,33,17> 0.0) -> (s? t:f=w284:fxp<+/-,33,17>)
    n166 = To Fixed-Point(fixed-point type=fxp<+/-,32,16> 0.0 ("f"), number=w284) -> (fixed-point=w283:fxp<+/-,32,16>)
  }
  n167 = for {
    N: 20 -> [_]
    tunnel: w25 -> [w299] mode=indexing
    tunnel: [w296] -> w24 mode=indexing
    border: u32 0 ("Timeout") -> [_]
    w303 = refnum<k21> "Memory-MLP_2_B_0"  # Memory
    n168 = To Fixed-Point(fixed-point type=fxp<+/-,32,16> 0.0 ("f"), number=w299) -> (fixed-point=w304:fxp<+/-,32,16>)
    n169 = feedback #11() -> (w302:u32)
    n170 = Increment(x=w302) -> (x+1=w301:u32)
    n171 = feedback-in #11(w301) -> ()
    n172 = xnode ("Memory Read")("Address"=w302, "Memory In"=w303) -> ("Data"=w300:fxp<+/-,32,16>)  [unwired: 1 out]
    n173 = Add(x=w304, y=w300) -> (x+y=w306:fxp<+/-,33,17>)
    n174 = Greater Than 0?(x=w306) -> (x > 0?=w308:bool)
    n175 = Select(t=w306, s=w308, f=fxp<+/-,33,17> 0.0) -> (s? t:f=w297:fxp<+/-,33,17>)
    n176 = To Fixed-Point(fixed-point type=fxp<+/-,32,16> 0.0 ("f"), number=w297) -> (fixed-point=w296:fxp<+/-,32,16>)
  }
  n177 = xnode ("FIFO Method Node")("Element"=w29, "Timeout"=0) -> ()  [unwired: 1 in, 2 out]
  n178 = call "Matrix*Vector2"("Vector b"=w6) -> ("Vector c"=w38:fxp<+/-,64,37>[])  [unwired: 10 in]
  n179 = call "Matrix*Vector4"("Vector b"=w24) -> ("Vector c"=w27:fxp<+/-,64,37>[])  [unwired: 10 in]
  n180 = Index Array(array=w38, index=0) -> (element=w13:fxp<+/-,64,37>)
  n181 = Index Array(array=w27, index=0) -> (element=w12:fxp<+/-,64,37>)
  n182 = xnode ("Register Read")("Register In"=w34) -> ("Data"=w33:fxp<+/-,32,16>)  [unwired: 1 out]
  n183 = xnode ("Register Read")("Register In"=w22) -> ("Data"=w21:fxp<+/-,32,16>)  [unwired: 1 out]
  n184 = Add(x=w13, y=w33) -> (x+y=w8:fxp<+/-,32,16>)
  "y(MLP1)" <- w8
  n185 = Add(x=w12, y=w21) -> (x+y=w7:fxp<+/-,32,16>)
  "y(MLP2)" <- w7
  n186 = xnode ("FIFO Method Node")("Element"=w8, "Timeout"=0) -> ()  [unwired: 1 in, 2 out]
  n187 = xnode ("FIFO Method Node")("Element"=w7, "Timeout"=0) -> ()  [unwired: 1 in, 2 out]
